vi "PiezAlyzer_sub_WaveTable.vi"(0 "Digital in":refnum<vi>, 1 "reference in":refnum<vi>, 2 "Amplitude (um)":dbl, 3 "1. Select Wave Form":T1(ring), 5 "Gain":dbl, 7 "reference 3":refnum<vi>, 9 "Plateau (ms)":dbl, 10 "Numeric":i32=20000, 11 "reference 4":refnum<vi>, 12 "reference 5":refnum<vi>, 13 "Period (ms)":dbl, 14 "Duty cycle (%)":dbl, 15 "File Path Control":path) -> (4 "Array":dbl[](array[numeric]))   [LabVIEW 2013]
uses:
  <vilib>/Utility/file.llb/Read From Spreadsheet File (DBL).vi
  <vilib>/measure/NI_MABase.lvlib
  <vilib>/Analysis/NI_AALBase.lvlib
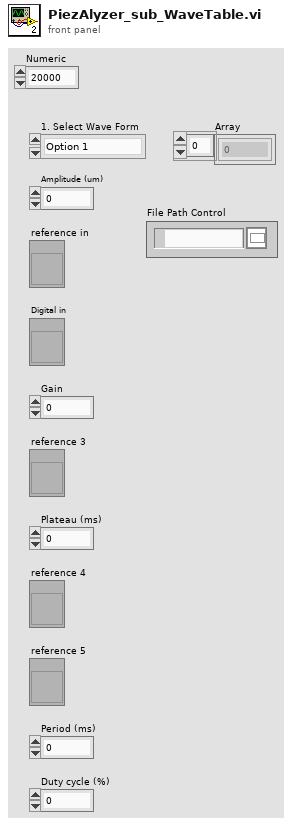
[diagram p1: front panel]
types:
  T1 = enum32{"Option 1", "Option 2", "Option 3", "Radio Selection 4", "Radio Selection 5", "From File"}
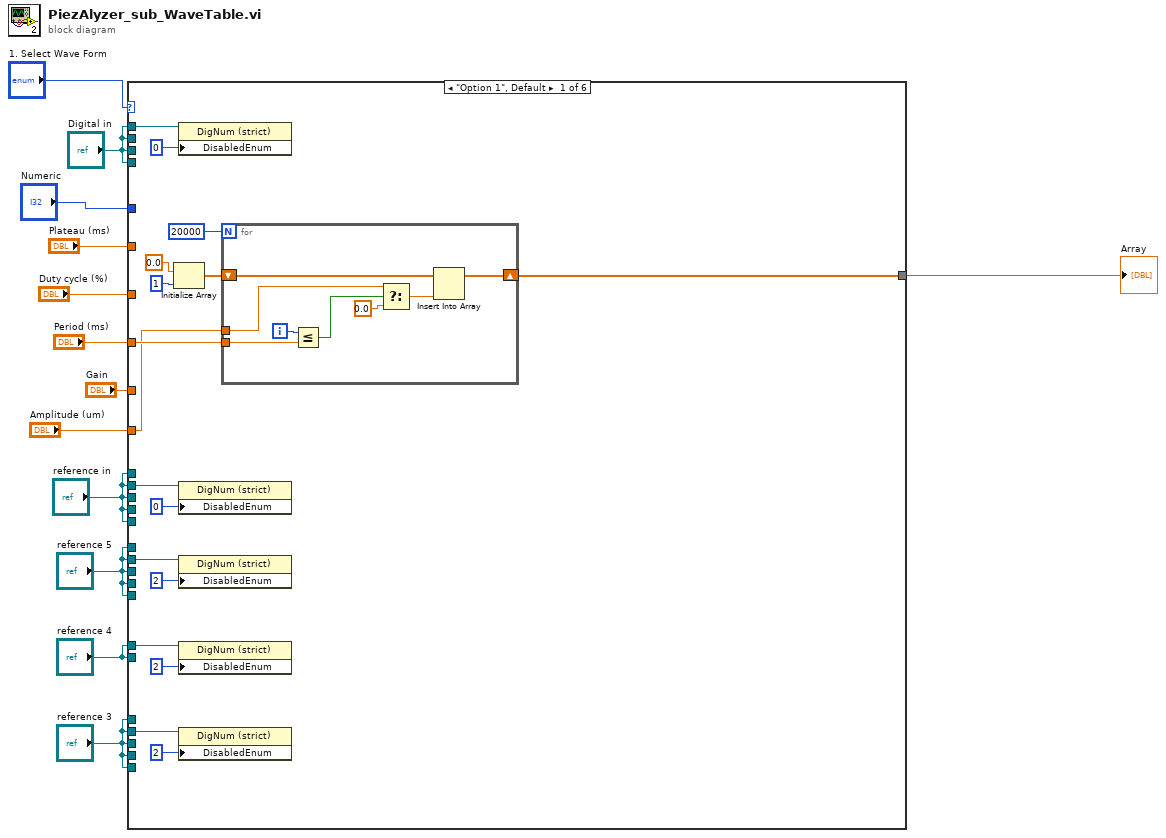
[diagram p0: block diagram]
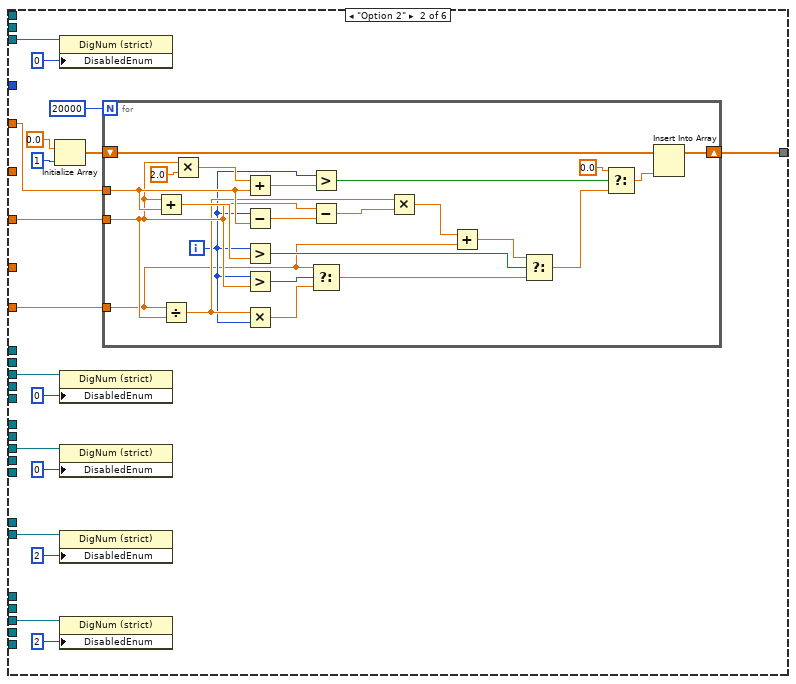
[diagram p2: hidden frame]
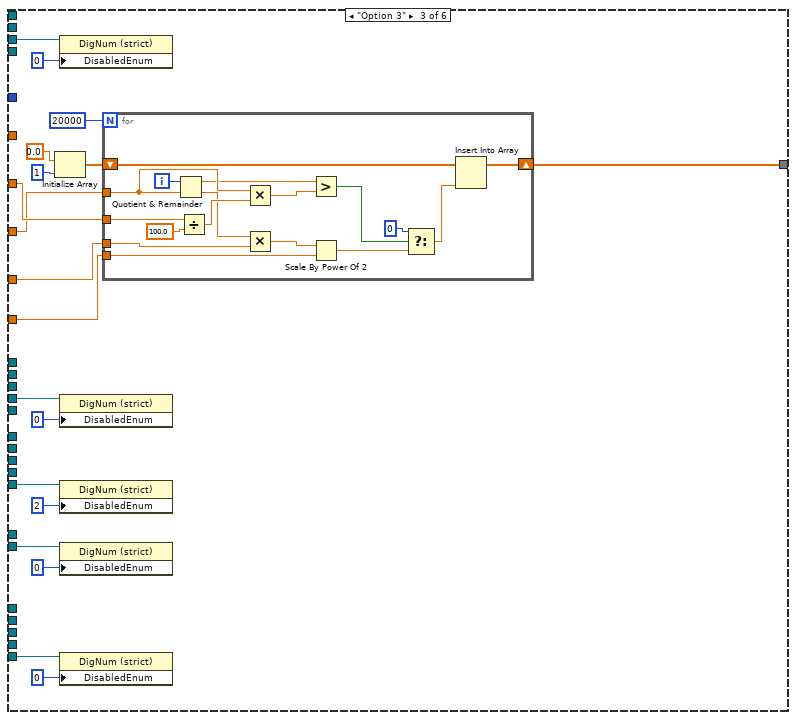
[diagram p3: hidden frame]
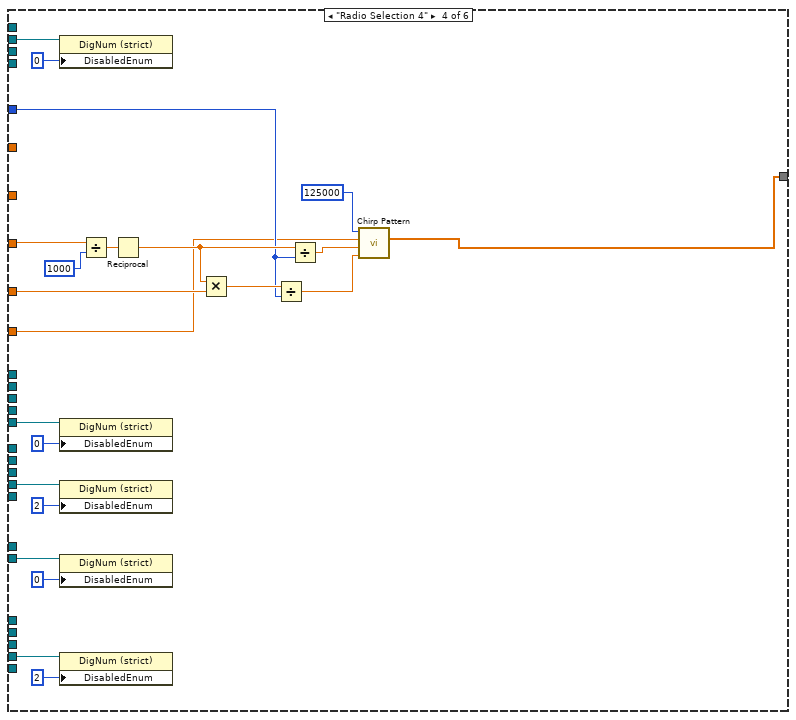
[diagram p4: hidden frame]
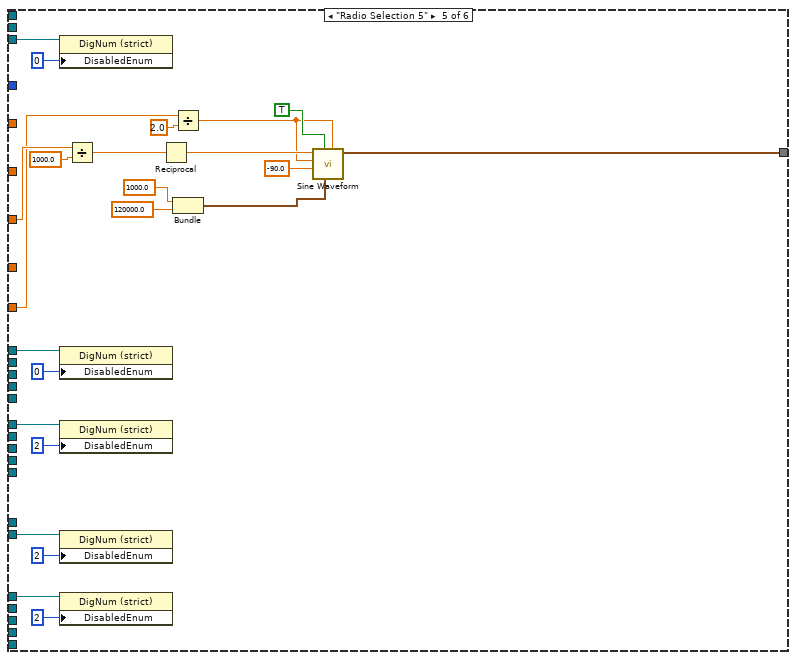
[diagram p5: hidden frame]
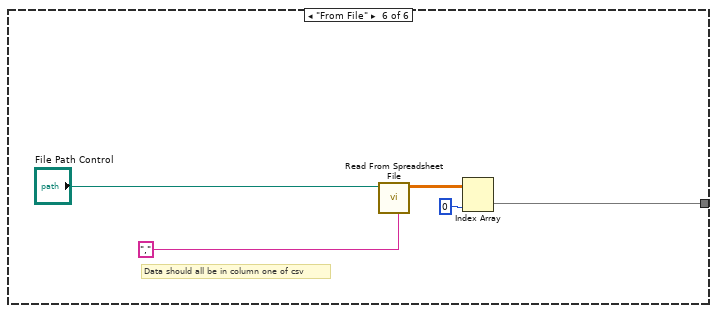
[diagram p6: hidden frame]
diagram:
  n1 = case shown="\"Option 1\", Default" "1. Select Wave Form" {
    tunnel: "Period (ms)" -> [w30 w55 w91 w127 w155 _]
    tunnel: "Duty cycle (%)" -> [_ _ w92 _ _ _]
    tunnel: "Amplitude (um)" -> [w29 w54 w93 w117 w145 _]
    tunnel: [w27 w49 w94 w116 w147 w163] -> w2
    tunnel: "Plateau (ms)" -> [_ w50 _ _ _ _]
    tunnel: "Gain" -> [_ _ w90 w124 _ _]
    tunnel: "Digital in" -> [w18 _ _ _ _ _]
    tunnel: "reference in" -> [w17 _ _ _ _ _]
    tunnel: "reference 3" -> [w16 _ _ _ _ _]
    tunnel: "reference 4" -> [w15 _ _ _ _ _]
    tunnel: "reference 5" -> [w14 _ _ _ _ _]
    tunnel: "reference in" -> [_ w42 _ _ _ _]
    tunnel: "reference 3" -> [_ w41 _ _ _ _]
    tunnel: "reference 5" -> [_ w40 _ _ _ _]
    tunnel: "Digital in" -> [_ _ w84 _ _ _]
    tunnel: "reference in" -> [_ _ w83 _ _ _]
    tunnel: "reference 3" -> [_ _ w82 _ _ _]
    tunnel: "reference 5" -> [_ _ w81 _ _ _]
    tunnel: "Digital in" -> [_ _ _ w132 _ _]
    tunnel: "reference in" -> [_ _ _ w131 _ _]
    tunnel: "reference 3" -> [_ _ _ w130 _ _]
    tunnel: "reference 5" -> [_ _ _ w129 _ _]
    tunnel: "Digital in" -> [_ w43 _ _ w142 _]
    tunnel: "reference in" -> [_ _ _ _ w141 _]
    tunnel: "reference 3" -> [_ _ _ _ w140 _]
    tunnel: "reference 5" -> [_ _ _ _ w139 _]
    tunnel: "reference 4" -> [_ w39 w80 w128 w138 _]
    tunnel: "Numeric" -> [_ _ _ w119 _ _]
    frame "Option 1", Default {
      n2 = Initialize Array(0.0, 1) -> (w26:dbl[])
      n3 = property on="Property Node" class="DigNum (strict)"(reference=w18, "DisabledEnum"=0) -> ()  [unwired: 1 in, 2 out]
      n4 = property on="Property Node" class="DigNum (strict)"(reference=w17, "DisabledEnum"=0) -> ()  [unwired: 1 in, 2 out]
      n5 = property on="Property Node" class="DigNum (strict)"(reference=w14, "DisabledEnum"=2) -> ()  [unwired: 1 in, 2 out]
      n6 = property on="Property Node" class="DigNum (strict)"(reference=w15, "DisabledEnum"=2) -> ()  [unwired: 1 in, 2 out]
      n7 = property on="Property Node" class="DigNum (strict)"(reference=w16, "DisabledEnum"=2) -> ()  [unwired: 1 in, 2 out]
      n8 = for {
        N: 20000 -> [_]
        tunnel: w30 -> [w31]
        tunnel: w29 -> [w37]
        shift-right: [w35] -> w27
        shift-left: w26 -> [w33]
        i -> [w34]
        n9 = Less Or Equal?(x=w34, y=w31) -> (x <= y?=w38:bool)
        n10 = Select(t=w37, s=w38, f=0.0) -> (s? t:f=w32:dbl)
        n11 = Insert Into Array(array=w33, new element=w32) -> (w35:dbl[])  [unwired: 1 in]
      }
    }
    frame "Option 2" {
      n12 = Initialize Array(0.0, 1) -> (w51:dbl[])
      n13 = property on="Property Node" class="DigNum (strict)"(reference=w43, "DisabledEnum"=0) -> ()  [unwired: 1 in, 2 out]
      n14 = property on="Property Node" class="DigNum (strict)"(reference=w42, "DisabledEnum"=0) -> ()  [unwired: 1 in, 2 out]
      n15 = property on="Property Node" class="DigNum (strict)"(reference=w40, "DisabledEnum"=0) -> ()  [unwired: 1 in, 2 out]
      n16 = property on="Property Node" class="DigNum (strict)"(reference=w39, "DisabledEnum"=2) -> ()  [unwired: 1 in, 2 out]
      n17 = property on="Property Node" class="DigNum (strict)"(reference=w41, "DisabledEnum"=2) -> ()  [unwired: 1 in, 2 out]
      n18 = for {
        N: 20000 -> [_]
        shift-right: [w79] -> w49
        shift-left: w51 -> [w78]
        tunnel: w55 -> [w63]
        tunnel: w54 -> [w58]
        tunnel: w50 -> [w68]
        i -> [w60]
        n19 = Add(x=w63, y=w68) -> (x+y=w71:dbl)
        n20 = Divide(x=w58, y=w63) -> (x/y=w61:dbl)
        n21 = Multiply(x=w63, y=2.0) -> (x*y=w76:dbl)
        n22 = Add(x=w76, y=w68) -> (x+y=w75:dbl)
        n23 = Subtract(x=w60, y=w68) -> (x-y=w67:dbl)
        n24 = Greater?(x=w60, y=w71) -> (0:w70:bool)
        n25 = Greater?(x=w60, y=w63) -> (0:w64:bool)
        n26 = Multiply(x=w61, y=w60) -> (x*y=w62:dbl)
        n27 = Greater?(x=w60, y=w75) -> (0:w74:bool)
        n28 = Subtract(x=w63, y=w67) -> (x-y=w66:dbl)
        n29 = Select(t=w58, s=w64, f=w62) -> (s? t:f=w65:dbl)
        n30 = Multiply(x=w61, y=w66) -> (x*y=w59:dbl)
        n31 = Add(x=w59, y=w58) -> (x+y=w57:dbl)
        n32 = Select(t=w57, s=w70, f=w65) -> (s? t:f=w69:dbl)
        n33 = Select(t=0.0, s=w74, f=w69) -> (s? t:f=w72:dbl)
        n34 = Insert Into Array(array=w78, new element=w72) -> (w79:dbl[])  [unwired: 1 in]
      }
    }
    frame "Option 3" {
      n35 = Initialize Array(0.0, 1) -> (w97:dbl[])
      n36 = property on="Property Node" class="DigNum (strict)"(reference=w84, "DisabledEnum"=0) -> ()  [unwired: 1 in, 2 out]
      n37 = property on="Property Node" class="DigNum (strict)"(reference=w83, "DisabledEnum"=0) -> ()  [unwired: 1 in, 2 out]
      n38 = property on="Property Node" class="DigNum (strict)"(reference=w81, "DisabledEnum"=2) -> ()  [unwired: 1 in, 2 out]
      n39 = property on="Property Node" class="DigNum (strict)"(reference=w80, "DisabledEnum"=0) -> ()  [unwired: 1 in, 2 out]
      n40 = property on="Property Node" class="DigNum (strict)"(reference=w82, "DisabledEnum"=0) -> ()  [unwired: 1 in, 2 out]
      n41 = for {
        N: 20000 -> [_]
        tunnel: w91 -> [w105]
        tunnel: w92 -> [w109]
        tunnel: w93 -> [w101]
        shift-right: [w115] -> w94
        shift-left: w97 -> [w114]
        tunnel: w90 -> [w103]
        i -> [w113]
        n42 = Quotient & Remainder(x=w113, y=w105) -> (x-y*floor(x/y)=w104:dbl, floor(x/y)=w102:dbl)
        n43 = Divide(x=w109, y=100.0) -> (x/y=w107:dbl)
        n44 = Multiply(x=w105, y=w107) -> (x*y=w106:dbl)
        n45 = Multiply(x=w102, y=w103) -> (x*y=w100:dbl)
        n46 = Greater?(x=w104, y=w106) -> (0:w112:bool)
        n47 = Scale By Power Of 2(n=w100, x=w101) -> (x*2^n=w99:dbl)
        n48 = Select(t=0, s=w112, f=w99) -> (s? t:f=w110:dbl)
        n49 = Insert Into Array(array=w114, new element=w110) -> (w115:dbl[])  [unwired: 1 in]
      }
    }
    frame "Radio Selection 4" {
      n50 = property on="Property Node" class="DigNum (strict)"(reference=w132, "DisabledEnum"=0) -> ()  [unwired: 1 in, 2 out]
      n51 = property on="Property Node" class="DigNum (strict)"(reference=w131, "DisabledEnum"=0) -> ()  [unwired: 1 in, 2 out]
      n52 = property on="Property Node" class="DigNum (strict)"(reference=w129, "DisabledEnum"=2) -> ()  [unwired: 1 in, 2 out]
      n53 = property on="Property Node" class="DigNum (strict)"(reference=w128, "DisabledEnum"=0) -> ()  [unwired: 1 in, 2 out]
      n54 = property on="Property Node" class="DigNum (strict)"(reference=w130, "DisabledEnum"=2) -> ()  [unwired: 1 in, 2 out]
      n55 = Divide(x=w127, y=1000) -> (x/y=w125:dbl)
      n56 = Reciprocal(x=w125) -> (1/x=w122:dbl)
      n57 = Multiply(x=w122, y=w124) -> (x*y=w123:dbl)
      n58 = Divide(x=w123, y=w119) -> (x/y=w120:dbl)
      n59 = Divide(x=w122, y=w119) -> (x/y=w121:dbl)
      n60 = call <vilib>:"Chirp Pattern.vi"("f2"=w120, "f1"=w121, "amplitude"=w117, "samples"=125000) -> ("Chirp Pattern"=w116:dbl[])  [unwired: 1 out]
    }
    frame "Radio Selection 5" {
      n61 = property on="Property Node" class="DigNum (strict)"(reference=w142, "DisabledEnum"=0) -> ()  [unwired: 1 in, 2 out]
      n62 = property on="Property Node" class="DigNum (strict)"(reference=w141, "DisabledEnum"=0) -> ()  [unwired: 1 in, 2 out]
      n63 = property on="Property Node" class="DigNum (strict)"(reference=w139, "DisabledEnum"=2) -> ()  [unwired: 1 in, 2 out]
      n64 = property on="Property Node" class="DigNum (strict)"(reference=w138, "DisabledEnum"=2) -> ()  [unwired: 1 in, 2 out]
      n65 = property on="Property Node" class="DigNum (strict)"(reference=w140, "DisabledEnum"=2) -> ()  [unwired: 1 in, 2 out]
      n66 = Divide(x=w155, y=1000.0) -> (x/y=w153:dbl)
      n67 = Reciprocal(x=w153) -> (1/x=w152:dbl)
      n68 = Divide(x=w145, y=2.0) -> (x/y=w144:dbl)
      n69 = Bundle(1000.0, 120000.0) -> (w148:cluster{dbl, dbl})  [unwired: 1 in]
      n70 = call <vilib>:"Sine Waveform.vi"("offset"=w144, "sampling info"=w148, "reset signal"=TRUE, "phase"=-90.0, "amplitude"=w144, "frequency"=w152) -> ("signal out"=w147:waveform(dbl))  [unwired: 4 in, 1 out]
    }
    frame "From File" {
      # "Data should all be in column one of csv"
      n71 = call-poly <vilib>:"Read From Spreadsheet File.vi"("delimiter (\\t)"="," ("delimiter (\\t)"), "file path (dialog if empty)"="File Path Control") -> ("all rows"=w164:dbl[][])  [unwired: 5 in, 4 out]
      n72 = Index Array(array=w164, index (col)=0 ("disabled index (col)")) -> (element=w163:dbl[])  [unwired: 1 in]
    }
  }
  "Array" <- w2
